vi "Scan_Hopping_IT_VUW.vi"() -> ()   [LabVIEW 2023]
uses:
  Sub_Vi/TypeDefs/Settings.ctl
  Sub_Vi/TypeDefs/ChangeOnFly.ctl
  Sub_Vi/TypeDefs/Display.ctl
  Settings.vi
panel:
  in  "Feedback Threshold \nUpper (Amps)":dbl=-1e-12
  in  "StopCond_GreaterThan? 2":bool
  in  "IT Time /s":dbl=10.0 format="%#_13g"
  in  "Display Cluster":T1
  in  "ChangeonFly":T2
  in  "SettingsCluster":T3={"Sample Rate (us)"=1, "Samples Per Data Point (int, power of 2)"=1000, "DistanceToBulk (um)"=-1.0, "HoldTimeScaler"=40000, "SaveData"=TRUE, "DistanceToBulk (um) 2"=-1.0, "DistanceToBulk (um) 3"=-1.0}
  in  "Feedback Type":T4(ring)=enum."Current 1"
  in  "StopCond_GreaterThan?":bool=TRUE
  in  "Approach Rate (um/s)":dbl=0.15
  in  "Retract Rate (um/s)":dbl=1.0
  in  "Hopping Distance (um)":dbl=1.0
  in  "Z End (um)":dbl
  in  "Distance To Retract (um)":dbl=5.0
  in  "Upper dZ limit":i32=8
  in  "Feedback Threshold \nLower  (Amps)":dbl=1e-12
  in  "P":fxp<+/-,32,1>=0.029999999795109034 format="%.32g"
  in  "X Center (um)":dbl=150.0 min=0.0 max=300.0
  in  "Y Center (um)":dbl=150.0 min=0.0 max=300.0
  in  "Y Width (um)":dbl=10.0
  in  "X Width (um)":dbl=10.0
  in  "Scan Rate (um/s)":dbl=5.0
  in  "Voltage to Electrode (V)":dbl=-0.4
  in  "IT Time Delta /s":dbl=0.5
  in  "Z Start height (um)":dbl=150.0
  in  "Start scan Button":bool
  in  "Stop":bool
  in  "Pause":bool
  in  "Start Scanning Button":bool
  out "Y end":dbl
  out "X end":dbl
  out "X start":dbl
  out "Y start":dbl
  in  "Tab Control 4":enum32{"AC Approach 2"}(tab)
  out "t vs C1":dbl[](graph)
  out "Z vs C1":cluster{"Y":dbl[], "Y":dbl[]}[](graph)
  # "Feedback  Settings"
  # "Approach  Settings"
  # "IT  Settings"
  # "Scan  Settings"
  # "Define Scan area \nAbout centre"
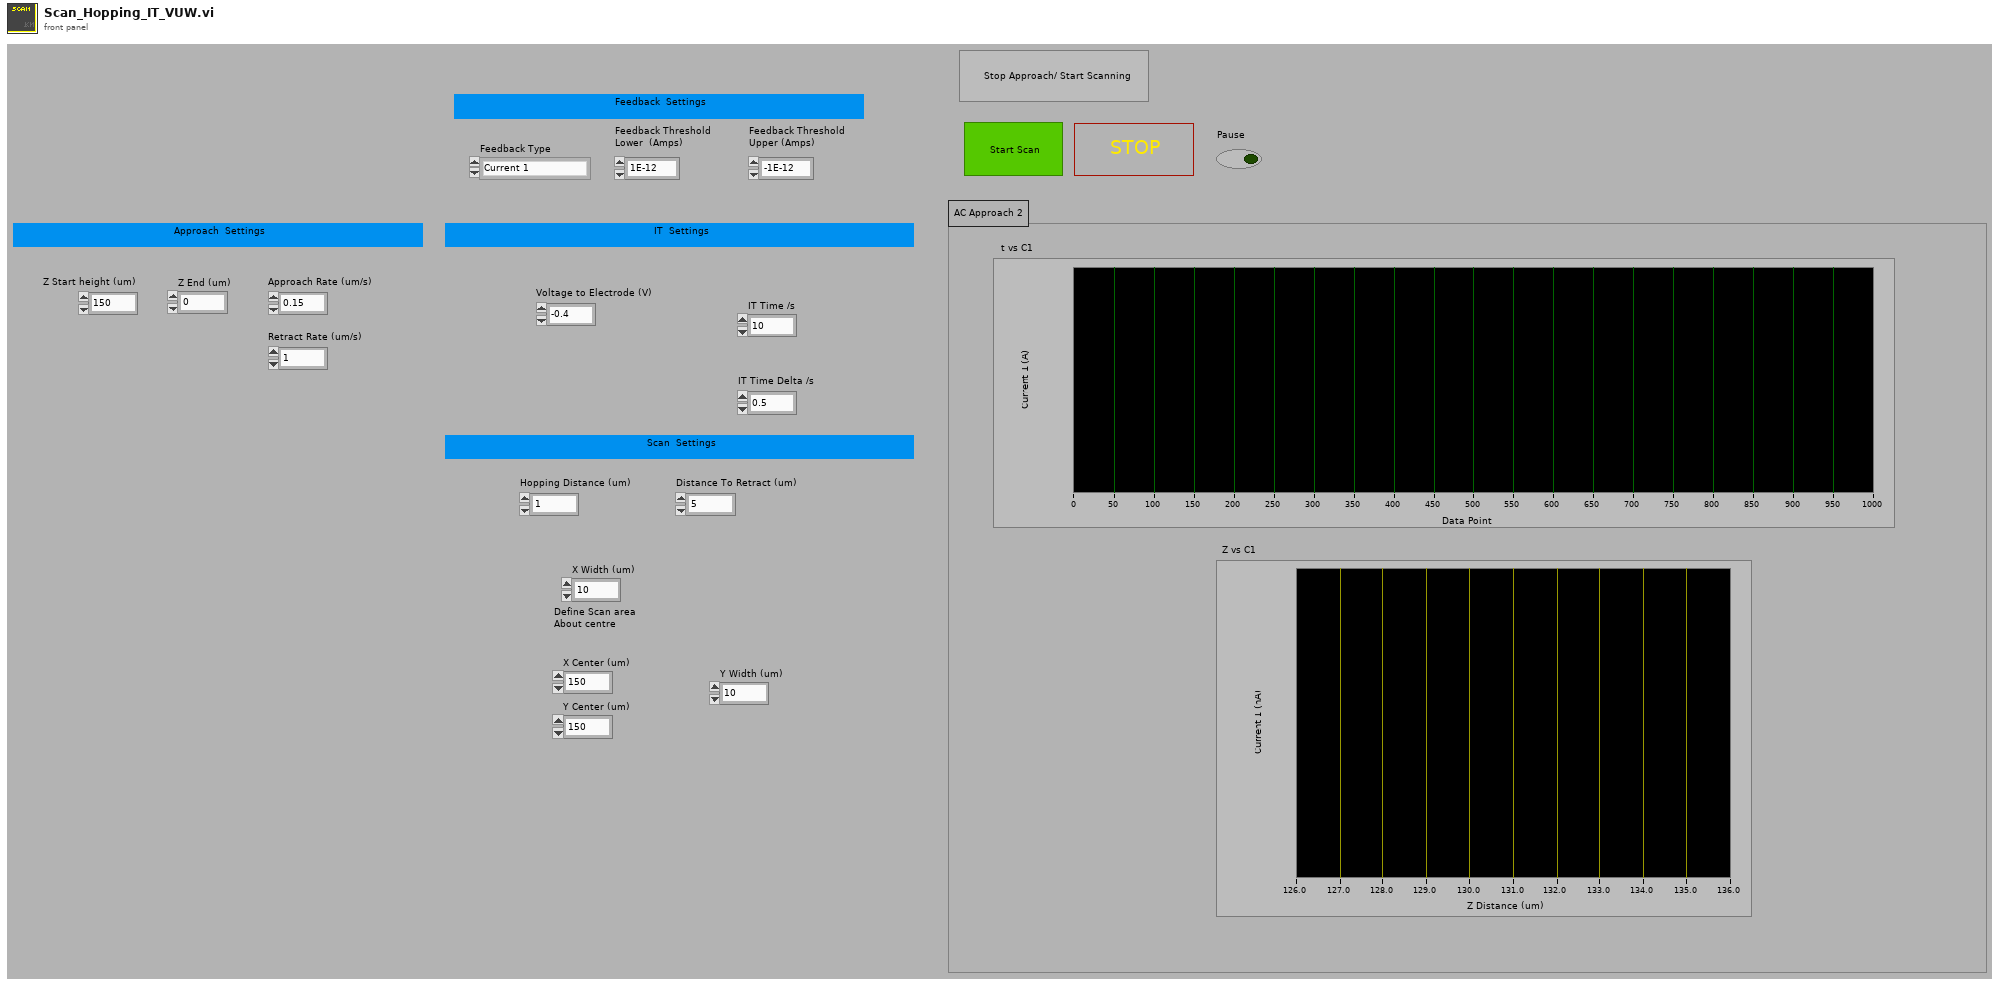
[diagram p1: front panel]
types:
  T1 = typedef "Display.ctl" = cluster{"X":refnum<vi>, "Y":refnum<vi>, "Z":refnum<vi>, "Amp":refnum<vi>, "Phase":refnum<vi>, "t vs Z":refnum<vi>, "t vs C1":refnum<vi>, "t vs C2":refnum<vi>, "t vs C3":refnum<vi>, "t vs Amp":refnum<vi>, "t vs Phase":refnum<vi>, "t vs X":refnum<vi>, "t vs Y":refnum<vi>, "Z vs C1":refnum<vi>, "Z vs C2":refnum<vi>, "Z vs C3":refnum<vi>, "V vs C1":refnum<vi>, "V vs C2":refnum<vi>, "V vs C3":refnum<vi>, "X/Y/Z F":refnum<vi>, "X/Y/Z R":refnum<vi>, "X/Y/C1 F":refnum<vi>, "X/Y/C1 R":refnum<vi>, "X/Y/C2 F":refnum<vi>, "X/Y/C2 R":refnum<vi>, "X/Y/C3 F":refnum<vi>, "X/Y/C3 R":refnum<vi>, "NumberOfLines":u16, "um Per Pixel":dbl, "um Per Line":dbl, "X Center":dbl, "Hop X/Y/Z":refnum<vi>, "Hop X/Y/C1":refnum<vi>, "Hop X/Y/C2":refnum<vi>, "Hop X/Y/C3":refnum<vi>, "X Width":dbl, "Y Width":dbl, "Hopping Distance":dbl, "V2 vs C1":refnum<vi>, "V vs Phase":refnum<vi>, "Y Center":dbl, "Number of Pixels":dbl, "V2 vs C2":refnum<vi>, "V2 vs C3":refnum<vi>, "V vs y":refnum<vi>, "V2 vs y":refnum<vi>, "Z vs Amp":refnum<vi>, "Z vs Phase":refnum<vi>}
  T2 = typedef "ChangeOnFly.ctl" = cluster{"Stop (boolean)":refnum<vi>, "Pause (boolean)":refnum<vi>, "EndCurrentLine (boolean)":refnum<vi>, "max movement per update step (Interger, nm)":refnum<vi>, "P (float, arb)":refnum<vi>, "Feedback set point (double, Amps)":refnum<vi>, "Voltage (double, V)":refnum<vi>, "Feedback set point 2 (double, Amps)":refnum<vi>, "Stop on Greater Than 2? (boolean)":refnum<vi>, "Stop on Greater Than? (boolean)":refnum<vi>, "Voltage 2 (double, V)":refnum<vi>, "Feedback Type (enum)":refnum<vi>, "Feedback Type 2 (enum)":refnum<vi>}
  T3 = typedef "Settings.ctl" = cluster{"Sample Rate (us)":u32, "Samples Per Data Point (int, power of 2)":i16, "DistanceToBulk (um)":dbl, "HoldTimeScaler":u64, "SaveData":bool, "DistanceToBulk (um) 2":dbl, "DistanceToBulk (um) 3":dbl}
  T4 = enum16{"AC Magnitude", "Current 1", "Current 2", "Phase"}
  T5 = cluster{"Scan Rate (um/s)":dbl, "X Start":dbl, "X End":dbl, "Y Start":dbl, "Y End":dbl, " Z Start":dbl, "HoppingDistance":dbl, "V":dbl, "Z End":dbl, "Approach Rate Hopping (um/s)":dbl, "Retrack Rate (um/s)":dbl, "V 2":dbl, "Approach Rate (um/s)":dbl, "Hold Time START / s":dbl, "Hold Time Delta / s":dbl, "Voltage to Electrode During Retract":dbl, "Pause on First Approach?":bool}
  T6 = typedef "WayPointCluster.ctl" = cluster{"X (um)":dbl[], "Y (um)":dbl[], "Z (um)":dbl[], "V (V)":dbl[], "X Velocity (um s-1)":dbl[], "Y Velocity (um s-1)":dbl[], "Z Velocity (um s-1)":dbl[], "V Velocity (V s-1)":dbl[], "FeedBack Type (enum)":u16[], "Move X (boolean)":bool[], "Move Y (boolean)":bool[], "Move Z (boolean)":bool[], "Move V (boolean)":bool[], "Jump V (boolean)":bool[], "Hold (boolean)":bool[], "Hold Time":u32[], "V2 (V)":dbl[], "Move V2":bool[], "V2 Velocity (V s-1)":dbl[], "Jump V2 (boolean)":bool[], "Update z Position delta (ms)":i16[], "Hold Feedback1":bool[], "Move Z PicoMotor":bool[], " Z PicoMotor Direction":bool[], "DIO0":bool[]}
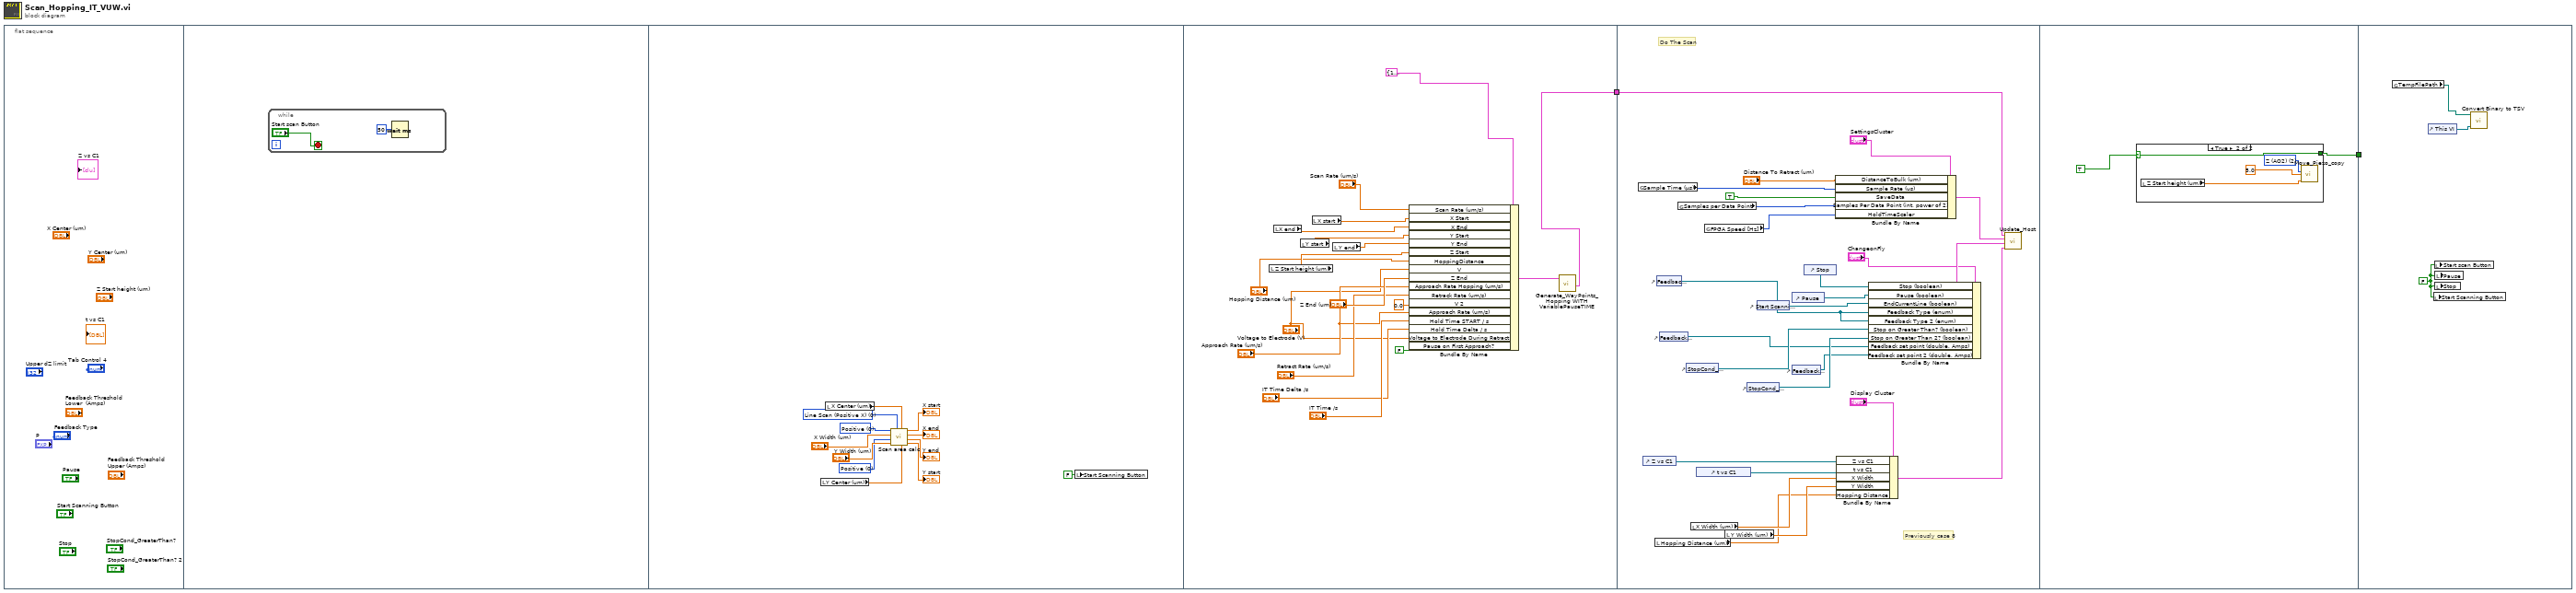
[diagram p0: block diagram]
diagram:
  n1 = flat-sequence {
    tunnel: [w34] -> w2
    tunnel: w2 -> [w59]
    tunnel: [w60] -> w1
    tunnel: w1 -> [_]
    frame #0 {
    }
    frame #1 {
      n2 = while {
        stop <- "Start scan Button" stop-if-true
        n3 = Wait (ms)(milliseconds to wait=u32 50) -> ()  [unwired: 1 out]
      }
    }
    frame #2 {
      w8 = u16 0 items=["Positive", "Negative"] ("Major Axis Direction")
      w7 = u16 0 items=["Positive", "Negative"] ("Minor Axis Direction")
      w6 = u16 0 items=["Line Scan (Positive X)", "Line Scan (Negative X)", "Line Scan (Positive Y)", "Line Scan (Negative Y)"] ("Scan Type")
      n4 = local read "Y Center (um)"() -> (w16:dbl)
      n5 = local read "X Center (um)"() -> (w15:dbl)
      n6 = call "Scan area calc.vi"("Y Width"="Y Width (um)", "Major Axis Direction"=w8, "X Width"="X Width (um)", "Minor Axis Direction"=w7, "Scan Type"=w6, "Y Center"=w16, "X Center"=w15) -> ("Y start"=→"Y start":dbl, "Y end"=→"Y end":dbl, "X end"=→"X end":dbl, "X start"=→"X start":dbl)
      n7 = local write "Start Scanning Button"(FALSE ("Start Scanning Button")) -> ()
    }
    frame #3 {
      n8 = local read "Z Start height (um)"() -> (w26:dbl)
      n9 = local read "X end"() -> (w29:dbl)
      n10 = local read "Y start"() -> (w28:dbl)
      n11 = local read "X start"() -> (w30:dbl)
      n12 = local read "Y end"() -> (w27:dbl)
      n13 = Bundle By Name(cluster=T5 {"Scan Rate (um/s)"=15.0, "X Start"=15.0, "X End"=15.0, "Y Start"=15.0, "Y End"=15.0, " Z Start"=15.0, "HoppingDistance"=1.0, "V"=15.0, "Z End"=15.0, "Approach Rate Hopping (um/s)"=15.0, "Retrack Rate (um/s)"=15.0, "V 2"=15.0, "Approach Rate (um/s)"=15.0, "Hold Time START / s"=15.0, "Hold Time Delta / s"=15.0, "Voltage to Electrode During Retract"=0.0, "Pause on First Approach?"=FALSE} ("Input Cluster"), "Scan Rate (um/s)"="Scan Rate (um/s)", "X Start"=w30, "X End"=w29, "Y Start"=w28, "Y End"=w27, "Z Start"=w26, "HoppingDistance"="Hopping Distance (um)", "V"="Voltage to Electrode (V)", "Z End"="Z End (um)", "Approach Rate Hopping (um/s)"="Approach Rate (um/s)", "Retrack Rate (um/s)"="Retract Rate (um/s)", "V 2"=0.0, "Approach Rate (um/s)"="Approach Rate (um/s)", "Hold Time START / s"="IT Time /s", "Hold Time Delta / s"="IT Time Delta /s", "Voltage to Electrode During Retract"="Voltage to Electrode (V)", "Pause on First Approach?"=FALSE) -> (w32:T5)
      n14 = call "Generate_WayPoints_Hopping WITH VariablePauseTIME.vi"("Input Cluster"=w32) -> ("output cluster"=w34:T6)  [unwired: 10 in]
    }
    frame #4 {
      # "Previously case 8"
      # "Do The Scan"
      n15 = global read "Settings.vi" "Sample Time (µs)"() -> (w42:u32)
      n16 = control-ref of="Z vs C1"() -> (w51:refnum<vi>)
      n17 = local read "Hopping Distance (um)"() -> (w48:dbl)
      n18 = control-ref of="Feedback Type"() -> (w40:refnum<vi>)
      n19 = control-ref of="Feedback Threshold \nLower  (Amps)"() -> (w37:refnum<vi>)
      n20 = global read "Settings.vi" "Samples per Data Point"() -> (w44:u16)
      n21 = control-ref of="StopCond_GreaterThan?"() -> (w39:refnum<vi>)
      n22 = local read "X Width (um)"() -> (w50:dbl)
      n23 = control-ref of="t vs C1"() -> (w52:refnum<vi>)
      n24 = global read "Settings.vi" "FPGA Speed [Hz]"() -> (w35:i64)
      n25 = local read "Y Width (um)"() -> (w49:dbl)
      n26 = control-ref of="StopCond_GreaterThan? 2"() -> (w38:refnum<vi>)
      n27 = control-ref of="Start Scanning Button"() -> (w55:refnum<vi>)
      n28 = control-ref of="Pause"() -> (w54:refnum<vi>)
      n29 = control-ref of="Feedback Threshold \nUpper (Amps)"() -> (w36:refnum<vi>)
      n30 = control-ref of="Stop"() -> (w53:refnum<vi>)
      n31 = Bundle By Name(cluster="SettingsCluster", "DistanceToBulk (um)"="Distance To Retract (um)", "Sample Rate (us)"=w42, "SaveData"=TRUE ("Save Data"), "Samples Per Data Point (int, power of 2)"=w44, "HoldTimeScaler"=w35) -> (w57:T3)
      n32 = Bundle By Name(cluster="Display Cluster", "Z vs C1"=w51, "t vs C1"=w52, "X Width"=w50, "Y Width"=w49, "Hopping Distance"=w48) -> (w58:T1)
      n33 = Bundle By Name(cluster="ChangeonFly", "Stop (boolean)"=w53, "Pause (boolean)"=w54, "EndCurrentLine (boolean)"=w55, "Feedback Type (enum)"=w40, "Feedback Type 2 (enum)"=w40, "Stop on Greater Than? (boolean)"=w39, "Stop on Greater Than 2? (boolean)"=w38, "Feedback set point (double, Amps)"=w37, "Feedback set point 2 (double, Amps)"=w36) -> (w56:T2)
      n34 = call "Update_Host.vi"("Display Cluster"=w58, "ChangeonFly"=w56, "SettingsCluster"=w57, "WayPointCluster"=w59) -> ()  [unwired: 6 in]
    }
    frame #5 {
      n35 = case shown="True" TRUE ("Retract after approach over (T/F)") {
        selector: TRUE ("Retract after approach over (T/F)") -> [w62 w63]
        tunnel: [w62 w63] -> w60
        frame False {
        }
        frame True {
          w66 = u16 2 items=["X (AO0)", "Y (AO1)", "Z (AO2)", "V (AO3)"] ("Channel")
          n36 = local read "Z Start height (um)"() -> (w64:dbl)
          n37 = call "Move_Piezo_copy.vi"("Piezo"=w66, "Movement Speed (µm/s)"=5.0 ("Scan Rate (um/s)"), "Position (µm) (or V)"=w64) -> ()  [unwired: 13 in]
        }
      }
    }
    frame #6 {
      w69 = FALSE ("Stop")
      n38 = global read "Settings.vi" "TempFilePath"() -> (w67:path)
      n39 = control-ref of="This VI"() -> (w68:refnum<vi>)
      n40 = local write "Start Scanning Button"(w69) -> ()
      n41 = local write "Start scan Button"(w69) -> ()
      n42 = local write "Pause"(w69) -> ()
      n43 = local write "Stop"(w69) -> ()
      n44 = call "Convert Binary to TSV.vi"("This VI"=w68, "TDMS DataFile Name"=w67) -> ()  [unwired: 10 in]
    }
  }
